vi "Create Execution Unit.vi"(8 "error in":errorcluster, 10 "Item Ref":T2=18446744073709551615 format="%.0x", 11 "Execution Unit Factory Implementation in":refnum<class "Execution Unit Factory Implementation.lvclass">) -> (0 "error out":errorcluster, 1 "Asynchronous Execution Units":T1[](array[typedef]) {"Outgoing Channels" format="%.0x"; "Incoming Channels" format="%.0x"}, 2 "Inline Execution Units":T1[](array[typedef]) {"Outgoing Channels" format="%.0x"; "Incoming Channels" format="%.0x"}, 3 "Execution Unit Factory Implementation out":refnum<class "Execution Unit Factory Implementation.lvclass">)   [LabVIEW 2020, in "Communication Bus Template Engine.lvlib" / "Implementation.lvlib" / "Execution Unit Factory Implementation.lvclass"]
uses:
  Execution Unit Factory Implementation.lvclass
  <vilib>/NI VeriStand/Custom Device API/Custom Device Item Ref.ctl
  Interfaces/Execution Unit/Execution Unit Information.ctl
  Interfaces/Execution Unit/Execution Unit/Execution Unit.lvclass
  Execution Unit Implementation/Execution Unit Implementation.lvclass
  C:/Dev/GitHub/niveristand-communications-bus-template/Source/Interfaces/Execution Unit/Execution Unit/Execution Unit.lvclass
  <vilib>/NI VeriStand/Custom Device API/Custom Device API.lvlib
  Interfaces/Interface.lvlib
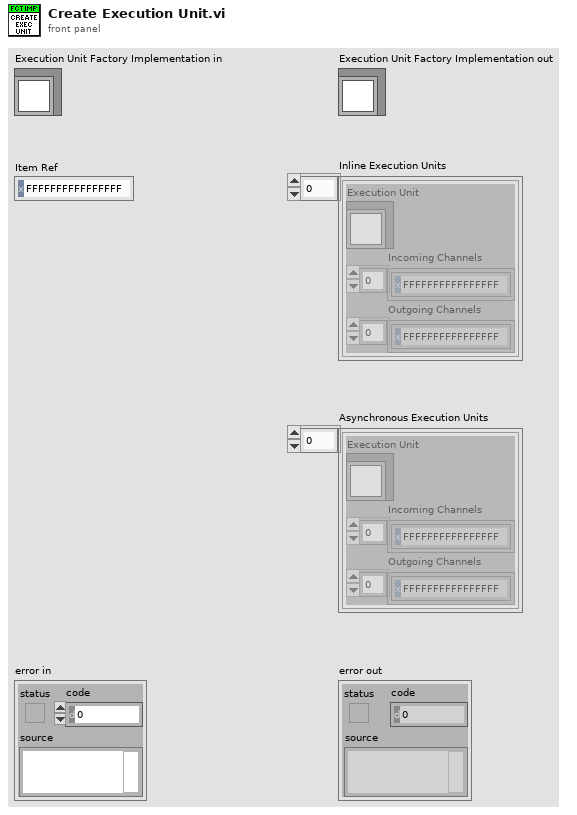
[diagram p1: front panel]
types:
  T1 = typedef "Communication Bus Template Engine.lvlib/Interface.lvlib/Execution Unit Information.ctl" = cluster{"Execution Unit":refnum<class "Execution Unit.lvclass">, "Incoming Channels":T2[], "Outgoing Channels":T2[]}
  T2 = typedef "Custom Device API.lvlib/Custom Device Item Ref.ctl" = u64
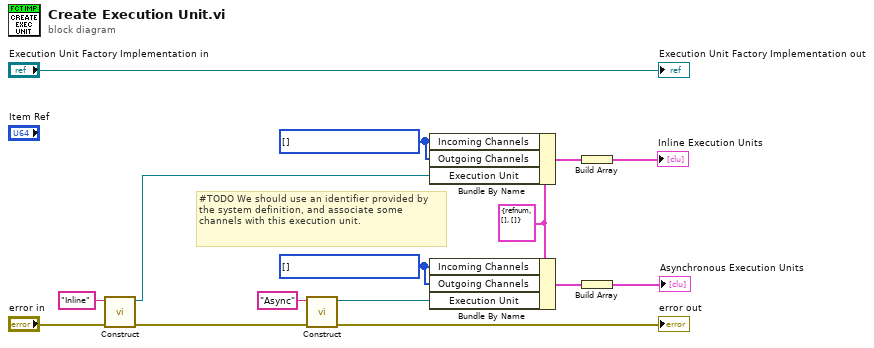
[diagram p0: block diagram]
diagram:
  w8 = T2[] [] ("Incoming Channels")
  w14 = T2[] [] ("Incoming Channels")
  w9 = T1 {"Execution Unit"=refnum, "Incoming Channels"=[], "Outgoing Channels"=[]} ("Execution Unit Information")
  # "#TODO We should use an identifier provided by the system definition, and associate some channels with this execution unit."
  n1 = call "Construct.vi"("error in (no error)"="error in", "id"="Inline") -> ("error out"=w4:errorcluster, "Execution Unit Implementation"=w3:refnum<class "Execution Unit Implementation.lvclass">)  [unwired: 8 in]
  n2 = call "Construct.vi"("error in (no error)"=w4, "id"="Async") -> ("error out"=→"error out":errorcluster, "Execution Unit Implementation"=w12:refnum<class "Execution Unit Implementation.lvclass">)  [unwired: 8 in]
  n3 = Bundle By Name(cluster=w9, "Incoming Channels"=w8, "Outgoing Channels"=w8, "Execution Unit"=w3) -> (w7:T1)
  n4 = Bundle By Name(cluster=w9, "Incoming Channels"=w14, "Outgoing Channels"=w14, "Execution Unit"=w12) -> (w11:T1)
  n5 = Build Array(w7) -> (→"Inline Execution Units":T1[])
  n6 = Build Array(w11) -> (→"Asynchronous Execution Units":T1[])
  "Execution Unit Factory Implementation out" <- "Execution Unit Factory Implementation in"
